vi "SortAccordingToXY.vi"(8 "error in (no error)":errorcluster, 11 "XYZ Point coordinates (pixels)":dbl[][](array[numeric])) -> (0 "error out":errorcluster, 3 "XYZ Point coordinates updated (pixels)":dbl[][](array[numeric]))   [LabVIEW 2010]
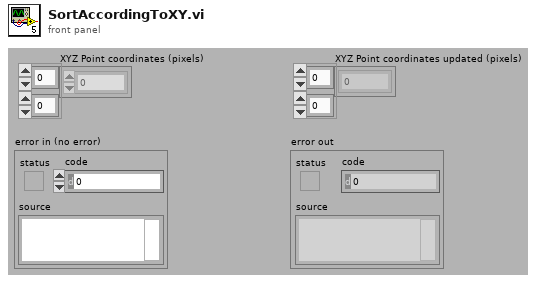
[diagram p1: front panel]
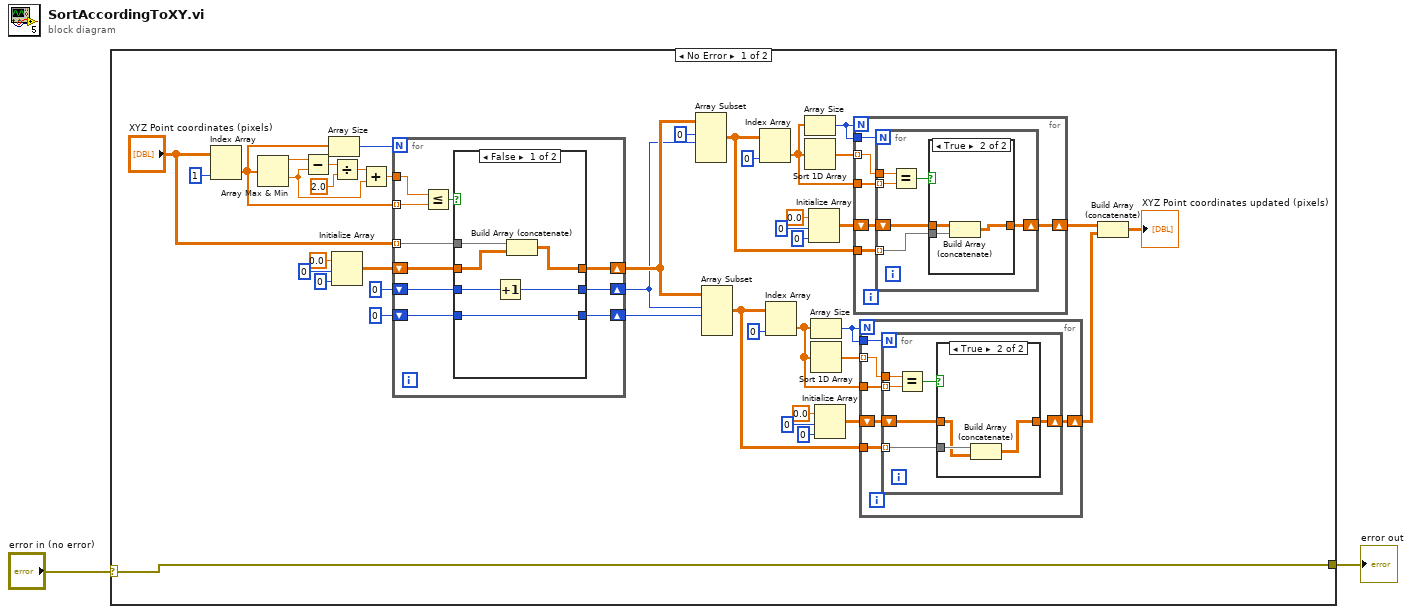
[diagram p0: block diagram]
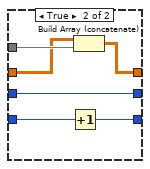
[diagram p4: hidden frame]
diagram:
  n1 = case shown="No Error" "error in (no error)" {
    selector: "error in (no error)" -> [w6 w99]
    tunnel: [w6 w99] -> w1
    frame No Error {
      n2 = Index Array(array="XYZ Point coordinates (pixels)", index (col)=1 ("disabled index (col)")) -> (element=w39:dbl[])  [unwired: 1 in]
      n3 = Array Max & Min(array=w39) -> (max value=w43:dbl, min value=w37:dbl)  [unwired: 2 out]
      n4 = Subtract(x=w43, y=w37) -> (x-y=w42:dbl)
      n5 = Array Size(array=w39) -> (size(s)=w40:i32)
      n6 = Divide(x=w42, y=2.0) -> (x/y=w38:dbl)
      n7 = Initialize Array(0.0 ("element"), 0 ("dimension size"), 0 ("dimension size")) -> (w32:dbl[][])
      n8 = Add(x=w38, y=w37) -> (x+y=w36:dbl)
      n9 = for {
        N: w40 -> [_]
        tunnel: w39 -> [w85] mode=indexing
        tunnel: "XYZ Point coordinates (pixels)" -> [w82] mode=indexing
        tunnel: w36 -> [w86]
        shift-right: [w81] -> w20
        shift-left: w32 -> [w83]
        shift-right: [w78] -> w4
        shift-left: 0 ("dimension size") -> [w80]
        shift-right: [w77] -> w19
        shift-left: 0 ("dimension size") -> [w79]
        n10 = Less Or Equal?(x=w86, y=w85) -> (x <= y?=w84:bool)
        n11 = case shown="False" w84 {
          tunnel: w83 -> [w91 w97]
          tunnel: w82 -> [w92 w98]
          tunnel: [w90 w96] -> w81
          tunnel: w80 -> [w89 w93]
          tunnel: w79 -> [w87 w95]
          tunnel: [w88 w93] -> w78
          tunnel: [w87 w94] -> w77
          frame False {
            n12 = Increment(x=w89) -> (x+1=w88:i32)
            n13 = Build Array (concatenate)(w92, w91) -> (w90:dbl[][])
          }
          frame True {
            n14 = Increment(x=w95) -> (x+1=w94:i32)
            n15 = Build Array (concatenate)(w97, w98) -> (w96:dbl[][])
          }
        }
      }
      n16 = Array Subset(array=w20, index (row)=0 ("index"), length (row)=w4) -> (w3:dbl[][])  [unwired: 2 in]
      n17 = Array Subset(array=w20, index (row)=w4, length (row)=w19) -> (w5:dbl[][])  [unwired: 2 in]
      n18 = Index Array(array=w3, index (col)=0 ("disabled index (col)")) -> (element=w23:dbl[])  [unwired: 1 in]
      n19 = Index Array(array=w5, index (col)=0 ("disabled index (col)")) -> (element=w13:dbl[])  [unwired: 1 in]
      n20 = Array Size(array=w23) -> (size(s)=w22:i32)
      n21 = Sort 1D Array(array=w23) -> (sorted array=w24:dbl[])
      n22 = Initialize Array(0.0 ("element"), 0 ("dimension size"), 0 ("dimension size")) -> (w21:dbl[][])
      n23 = Array Size(array=w13) -> (size(s)=w12:i32)
      n24 = Sort 1D Array(array=w13) -> (sorted array=w14:dbl[])
      n25 = Initialize Array(0.0 ("element"), 0 ("dimension size"), 0 ("dimension size")) -> (w11:dbl[][])
      n26 = for {
        N: w22 -> [_]
        tunnel: w24 -> [w66] mode=indexing
        tunnel: w23 -> [w65]
        tunnel: w3 -> [w64]
        tunnel: w22 -> [w63]
        shift-right: [w61] -> w7
        shift-left: w21 -> [w62]
        n27 = for {
          N: w63 -> [_]
          tunnel: w66 -> [w72]
          tunnel: w65 -> [w71] mode=indexing
          tunnel: w64 -> [w69] mode=indexing
          shift-right: [w67] -> w61
          shift-left: w62 -> [w68]
          n28 = Equal?(x=w72, y=w71) -> (x = y?=w70:bool)
          n29 = case shown="True" w70 {
            tunnel: w69 -> [_ w74]
            tunnel: w68 -> [w73 w75]
            tunnel: [w73 w76] -> w67
            frame False {
            }
            frame True {
              n30 = Build Array (concatenate)(w75, w74) -> (w76:dbl[][])
            }
          }
        }
      }
      n31 = for {
        N: w12 -> [_]
        tunnel: w14 -> [w50] mode=indexing
        tunnel: w13 -> [w49]
        tunnel: w5 -> [w48]
        tunnel: w12 -> [w47]
        shift-right: [w45] -> w10
        shift-left: w11 -> [w46]
        n32 = for {
          N: w47 -> [_]
          tunnel: w50 -> [w56]
          tunnel: w49 -> [w55] mode=indexing
          tunnel: w48 -> [w53] mode=indexing
          shift-right: [w51] -> w45
          shift-left: w46 -> [w52]
          n33 = Equal?(x=w56, y=w55) -> (x = y?=w54:bool)
          n34 = case shown="True" w54 {
            tunnel: w53 -> [_ w59]
            tunnel: w52 -> [w57 w58]
            tunnel: [w57 w60] -> w51
            frame False {
            }
            frame True {
              n35 = Build Array (concatenate)(w59, w58) -> (w60:dbl[][])
            }
          }
        }
      }
      n36 = Build Array (concatenate)(w7, w10) -> (→"XYZ Point coordinates updated (pixels)":dbl[][])
    }
    frame Error {
    }
  }
  "error out" <- w1
